vi "report_close.vi"(8 "error in (no error)":errorcluster, 11 "Instrument in":refnum<class "Instrument.lvclass">) -> (0 "error out":errorcluster, 3 "Instrument out":refnum<class "Instrument.lvclass">)   [LabVIEW 2019, in "Instrument.lvclass"]
uses:
  Instrument.lvclass
  Instrument.lvclass/Instrument.ctl
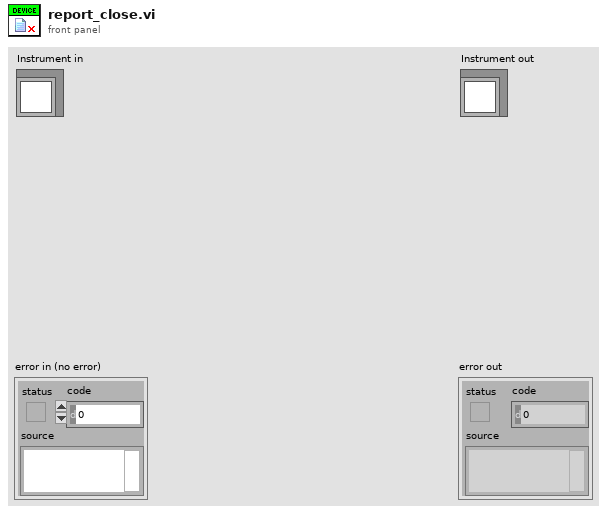
[diagram p1: front panel]
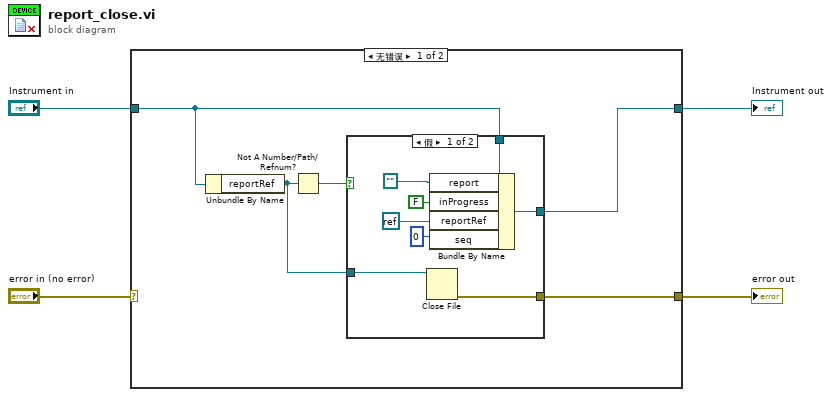
[diagram p0: block diagram]
diagram:
  n1 = case shown="无错误" "error in (no error)" {
    selector: "error in (no error)" -> [_ w20]
    tunnel: [w5 w20] -> w3
    tunnel: [w7 w19] -> w1
    tunnel: "Instrument in" -> [w8 w19]
    frame No Error {
      n2 = Unbundle By Name(w8) -> ("reportRef"=w6:refnum<file>)
      n3 = Not A Number/Path/Refnum?(number/path/refnum=w6) -> (NaN/Path/Refnum?=w9:bool)
      n4 = case shown="假" w9 {
        tunnel: w8 -> [w17 w18]
        tunnel: [w16 w18] -> w7
        tunnel: w6 -> [w11 _]
        tunnel: [w10 _] -> w5
        frame False {
          n5 = Close File(refnum=w11) -> (error out=w10:errorcluster)  [unwired: 1 in, 1 out]
          n6 = Bundle By Name(cluster=w17, "report"=path "", "inProgress"=FALSE, "reportRef"=refnum<k0> refnum, "seq"=0) -> (w16:refnum<class "Instrument.lvclass">)
        }
        frame True {
        }
      }
    }
    frame Error {
    }
  }
  "error out" <- w3
  "Instrument out" <- w1
